vi "02 Tools, Colors, and Clicks.vi"() -> ()   [LabVIEW 2019]
uses:
  _Subs/OpenDiagram/Open_XControl.xctl
panel:
  in  "OpenDiag":refnum<vi>(xcontrol)
  in  "stop":bool
  out "Waveform Chart":dbl(graph)
  in  "Slide":dbl(slide)=5.204081632653061 scale=0.0..10.0
  # "02 Tools, Colors, and Clicks\nThis code takes the value of the Slide and plots it - giving you a chance to try changing colors, ranges, etc.\n\nInstructions:\n1. Go to View:Tools Palette to bring it up\n2. hover over the tools and see what they all do.  Use the paint tool to change the color of the Chart and Slide\n3. Hit Run\n4. Click on the Axis Labels to edit\n5. Click on the lowest / highest value of the axis to rescale \n6. Right-btn click on the plot and select Properties - and edit..."
  # "Tools Palette"
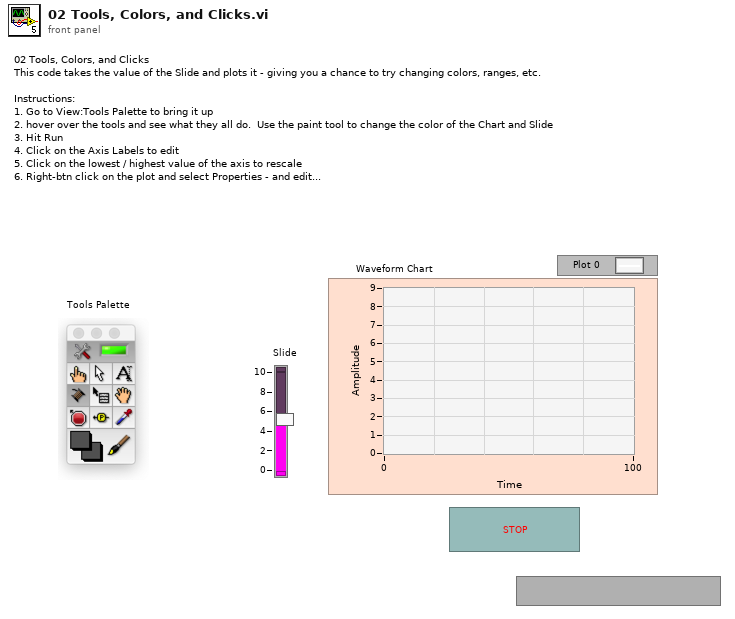
[diagram p1: front panel]
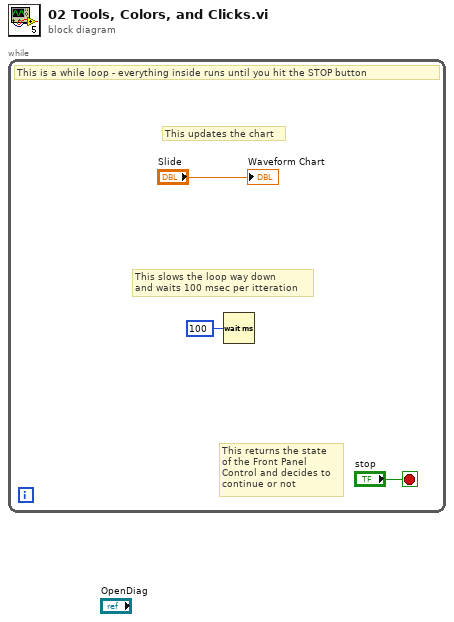
[diagram p0: block diagram]
diagram:
  n1 = while {
    stop <- "stop" stop-if-true
    # "This returns the state\nof the Front Panel \nControl and decides to\ncontinue or not"
    # "This slows the loop way down \nand waits 100 msec per itteration"
    # "This updates the chart"
    # "This is a while loop - everything inside runs until you hit the STOP button"
    n2 = Wait (ms)(milliseconds to wait=u32 100) -> ()  [unwired: 1 out]
    "Waveform Chart" <- "Slide"
  }
